vi "ISX3_Cmd_StartMeasure.vi"(1 "Number of Spectra":u16, 2 "Start/Stop":bool) -> (0 "Start/Stop measurement cmd":u8[](array[numeric]))   [LabVIEW 2012, in "Sciospec ISX3 Impedance Analyzer.lvlib"]
uses:
  Sciospec ISX3 Impedance Analyzer.lvlib
panel:
  # "This VI generates the command to start or stopp the measurement of a  the configured setup."
  # "If \"Number of Spectra\" equals '0' the measurement \nonly stops after the stop measurement command.\nIn any other case the measurement automatically stops."
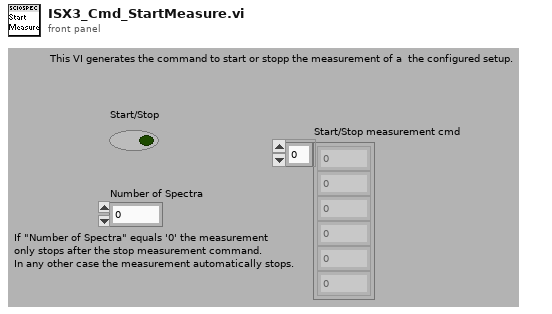
[diagram p1: front panel]
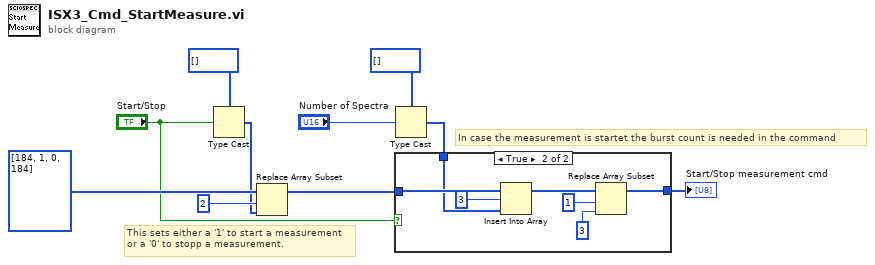
[diagram p0: block diagram]
diagram:
  # "In case the measurement is startet the burst count is needed in the command"
  # "This sets either a '1' to start a measurement\nor a '0' to stopp a measurement."
  n1 = Type Cast(type=u8[] [], x="Start/Stop") -> (*(type *) &x=w5:u8[])
  n2 = Replace Array Subset(array=u8[] [184, 1, 0, 184], new element=w5, index=2) -> (w3:u8[])
  n3 = Type Cast(type=u8[] [], x="Number of Spectra") -> (*(type *) &x=w2:u8[])
  n4 = case shown="True" "Start/Stop" {
    tunnel: w3 -> [w11 w17]
    tunnel: w2 -> [_ w16]
    tunnel: [w11 w12] -> w1
    frame False {
    }
    frame True {
      n5 = Insert Into Array(array=w17, index=3, new element=w16) -> (w13:u8[])
      n6 = Replace Array Subset(array=w13, new element=3, index=1) -> (w12:u8[])
    }
  }
  "Start/Stop measurement cmd" <- w1
